vi "Drive at Angle.vi"(4 "end power":dbl, 6 "Begin power":dbl, 8 "error in (no error)":errorcluster, 9 "Angle":dbl, 10 "Distance":dbl, 11 "RobotDriveDevRef":T1={"DevStatus"={"status"=FALSE, "code"=0, "source"=""}, "Motors[]"=[], "Square Inputs"=FALSE, "Max Output"=1.0}) -> (0 "error out":errorcluster, 1 "power out":dbl, 3 "refnum":T1={"DevStatus"={"status"=FALSE, "code"=0, "source"=""}, "Motors[]"=[], "Square Inputs"=FALSE, "Max Output"=1.0})   [LabVIEW 2019]
uses:
  <vilib>/Rock Robotics/WPI/RobotDrive/WPI_RobotDriveArcadeDrive_Standard(NoSaturation).vi
  Infinite Recharge current/Robot Global Data.vi
  <vilib>/Rock Robotics/WPI/ThirdParty/Phoenix-LabVIEW/Motor Controller/Get/CTRE_Phoenix_MotorController_GetSelectedSensorData.vi
  <vilib>/Rock Robotics/SystemInterfaces/DIO/FPGA_DIOPWMChannel.ctl
  <vilib>/Rock Robotics/WPI/PWM/WPI_PWMDeadband.ctl
  <vilib>/Rock Robotics/WPI/MotorControl/WPI_MotorControlType.ctl
  <vilib>/Rock Robotics/SystemInterfaces/DIO/FPGA_DIOChannel.ctl
  <vilib>/Rock Robotics/WPI/MotorControl/WPI_MotorControlDeviceRef.ctl
  <vilib>/Rock Robotics/WPI/RobotDrive/WPI_RobotDriveDevRef.ctl
panel:
  out "error":dbl
  out "x/y":dbl
  out "Distance Left 2":dbl format="%#_13g"
  out "rampdown":dbl format="%#_13g"
  out "Maximup":dbl format="%#_13g"
  out "rampup":dbl format="%#_13g"
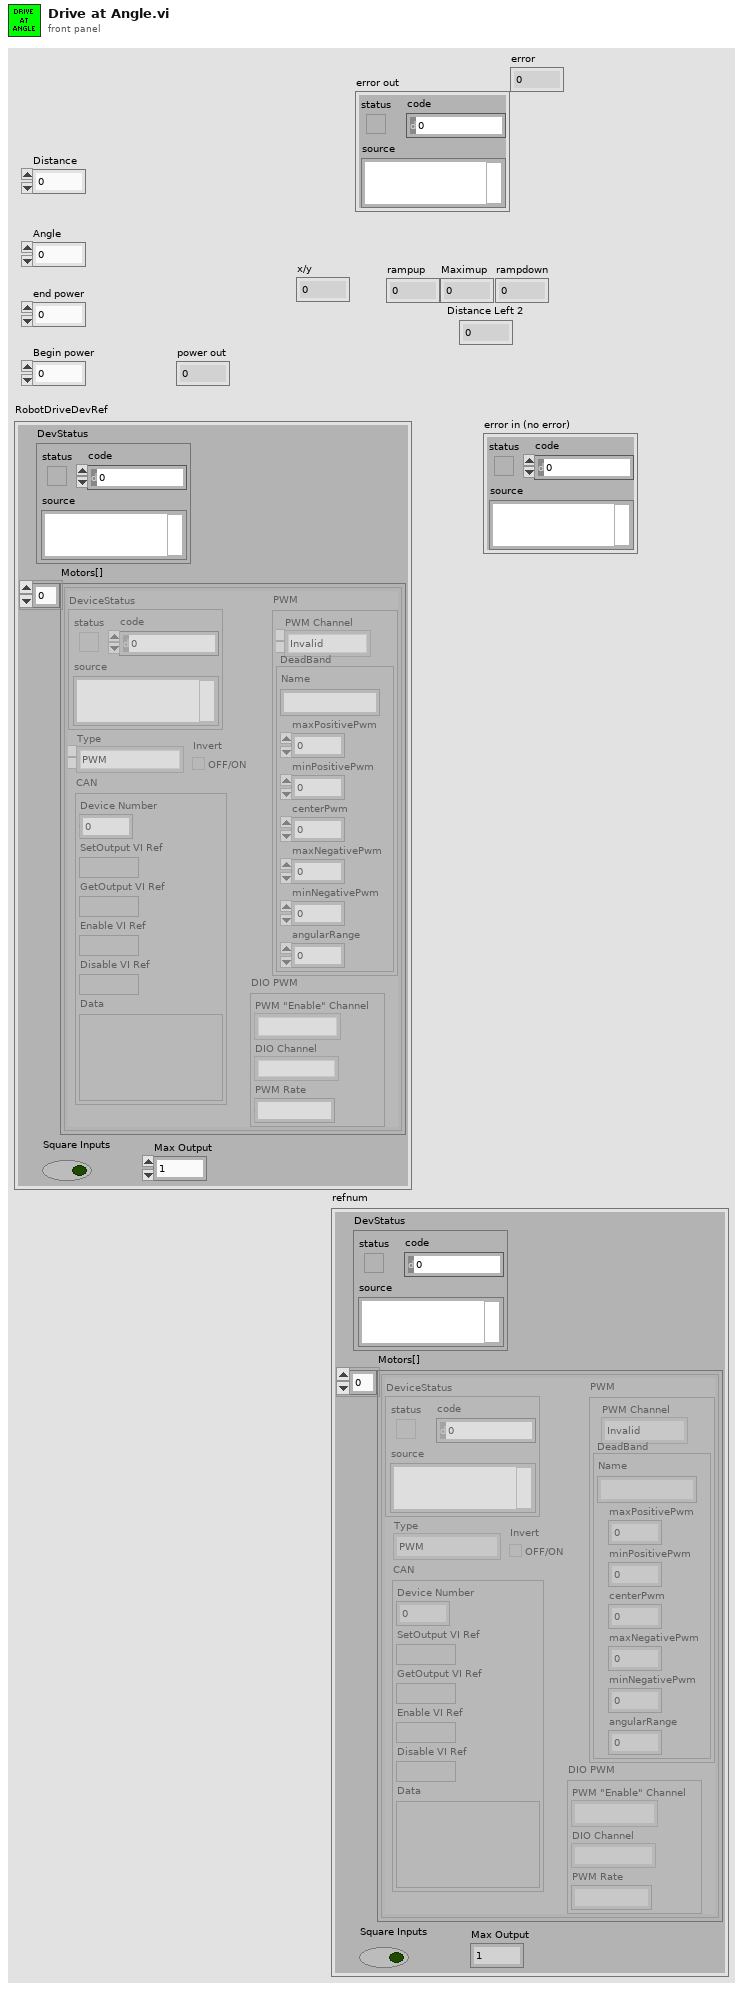
[diagram p1: front panel]
types:
  T1 = typedef "WPI_RobotDriveDevRef.ctl" = cluster{"DevStatus":errorcluster, "Motors[]":T2[], "Square Inputs":bool, "Max Output":dbl}
  T2 = typedef "WPI_MotorControlDeviceRef.ctl" = cluster{"DeviceStatus":errorcluster, "Type":T3, "PWM":cluster{"PWM Channel":T4, "DeadBand":T5}, "CAN":cluster{"Device Number":u8, "SetOutput VI Ref":variant, "GetOutput VI Ref":variant, "Enable VI Ref":variant, "Disable VI Ref":variant, "Data":variant}, "Invert":bool, "DIO PWM":cluster{"PWM \"Enable\" Channel":T4, "DIOChannel":T6, "PWM Rate":dbl}}
  T3 = typedef "WPI_MotorControlType.ctl" = enum16{"PWM", "CAN", "DIO PWM"}
  T4 = typedef "FPGA_DIOPWMChannel.ctl" = enum8{"PWM 0", "PWM 1", "PWM 2", "PWM 3", "PWM 4", "PWM 5", "PWM 6", "PWM 7", "PWM 8", "PWM 9", "PWM MXP 0", "PWM MXP 1", "PWM MXP 2", "PWM MXP 3", "PWM MXP 4", "PWM MXP 5", "PWM MXP 6", "PWM MXP 7", "PWM MXP 8", "PWM MXP 9", "Invalid"}
  T5 = typedef "WPI_PWMDeadband.ctl" = cluster{"Name":string, "maxPositivePwm":i32, "minPositivePwm":i32, "centerPwm":i32, "maxNegativePwm":i32, "minNegativePwm":i32, "angularRange":u16}
  T6 = typedef "FPGA_DIOChannel.ctl" = enum8{"DIO 0", "DIO 1", "DIO 2", "DIO 3", "DIO 4", "DIO 5", "DIO 6", "DIO 7", "DIO 8", "DIO 9", "DIO MXP 0", "DIO MXP 1", "DIO MXP 2", "DIO MXP 3", "DIO MXP 4", "DIO MXP 5", "DIO MXP 6", "DIO MXP 7", "DIO MXP 8", "DIO MXP 9", "DIO MXP 10", "DIO MXP 11", "DIO MXP 12", "DIO MXP 13", "DIO MXP 14", "DIO MXP 15", "SPI Port CS1", "SPI Port CS2", "SPI Port CS3", "SPI Port MISO", "SPI Port MOSI", "Invalid"}
  T7 = cluster{"Yaw":dbl, "Roll":dbl, "Pitch":dbl, "Heading":dbl, "Fused Heading":dbl}
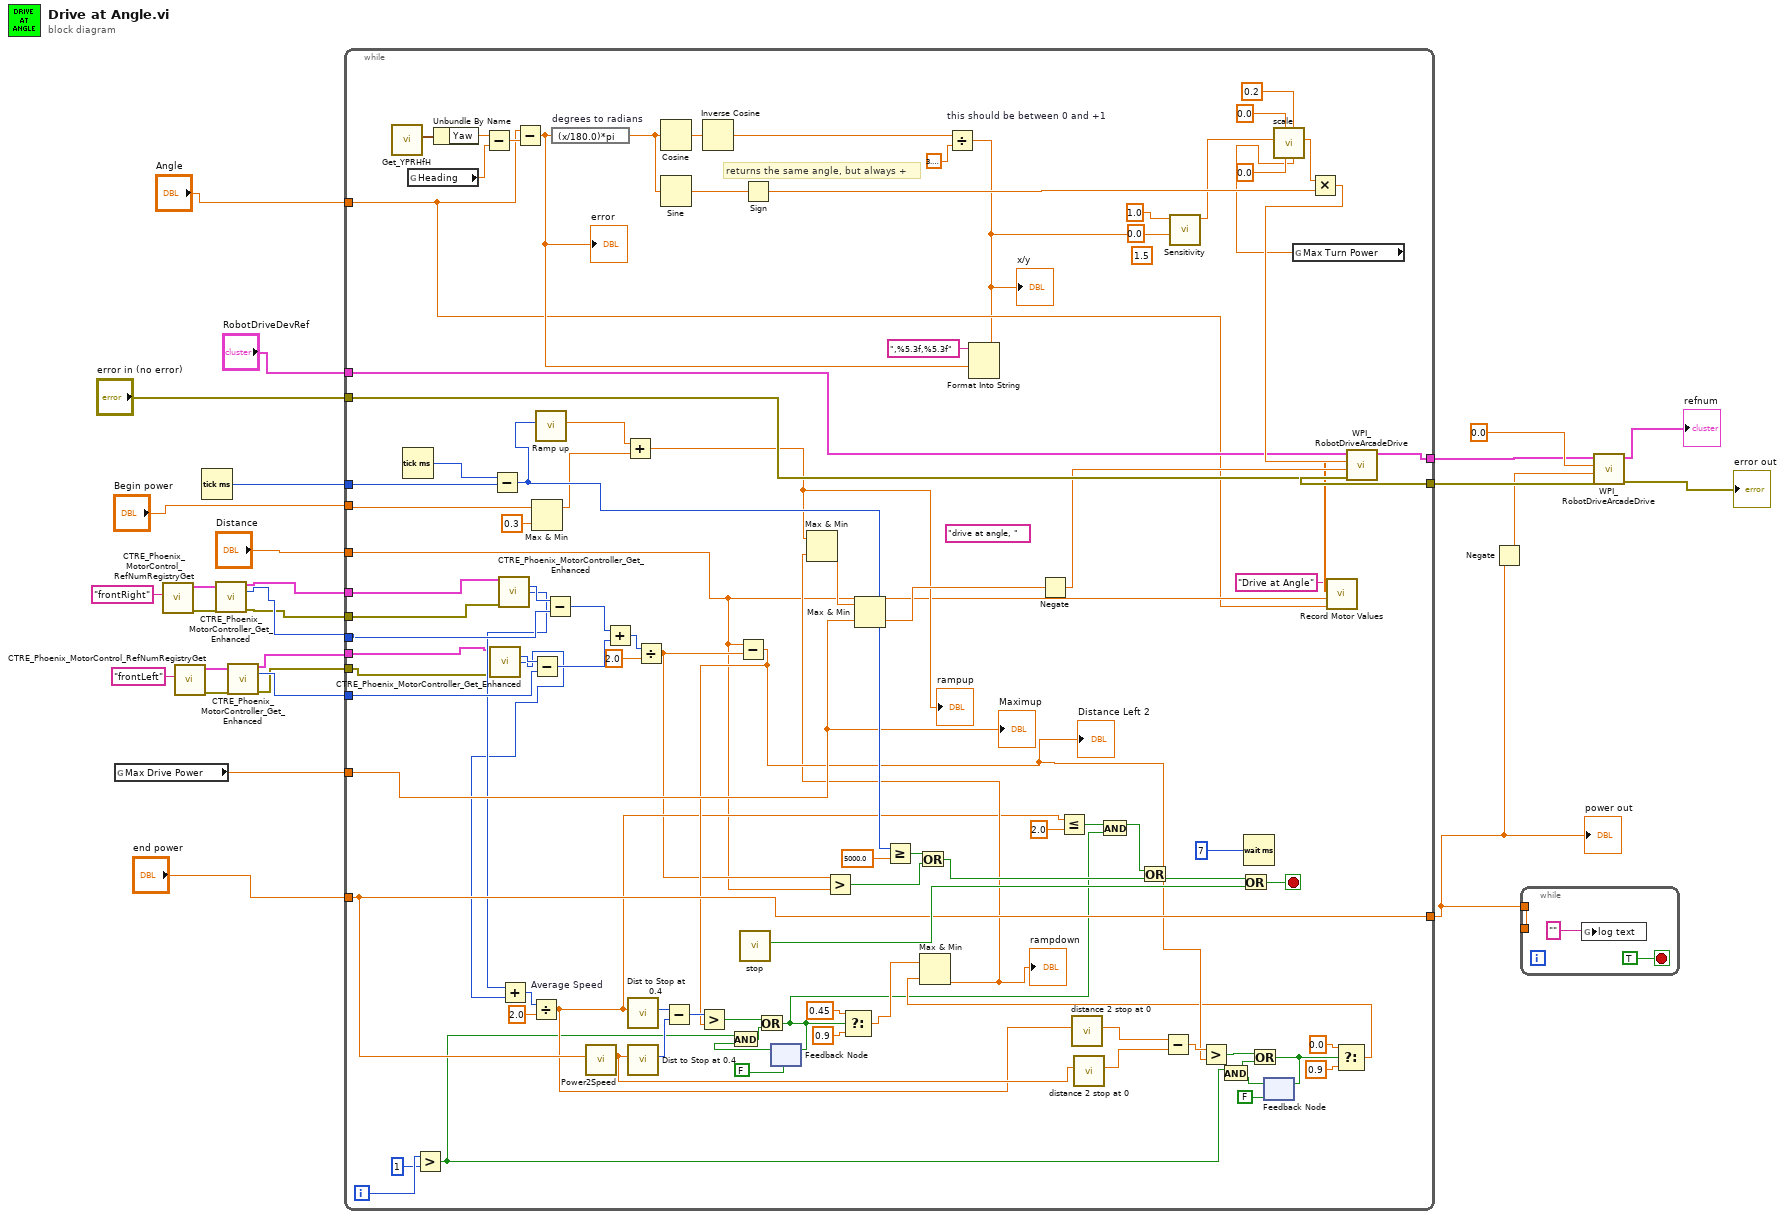
[diagram p0: block diagram]
diagram:
  n1 = global read "Robot Global Data.vi" "Max Drive Power"() -> (w15:dbl)
  n2 = call <vilib>:"CTRE_Phoenix_MotorControl_RefNumRegistryGet.vi"("refnum name"="frontRight") -> ("error out"=w7:errorcluster, "PhoenixMotorControlDevRef"=w8:T2)  [unwired: 9 in]
  n3 = call <vilib>:"CTRE_Phoenix_MotorControl_RefNumRegistryGet.vi"("refnum name"="frontLeft") -> ("error out"=w11:errorcluster, "PhoenixMotorControlDevRef"=w12:T2)  [unwired: 9 in]
  n4 = Tick Count (ms)() -> (millisecond timer value=w24:u32)
  n5 = call-poly <vilib>:"CTRE_Phoenix_MotorController_Get_Enhanced.vi"("PhoenixMotorControlDevRef"=w8, "error in"=w7) -> ("PhoenixMotorControlDevRef"=w4:T2, "Position (Raw Sensor Units)"=w5:i32, "error out"=w3:errorcluster)  [unwired: 10 in, 1 out]
  n6 = call-poly <vilib>:"CTRE_Phoenix_MotorController_Get_Enhanced.vi"("PhoenixMotorControlDevRef"=w12, "error in"=w11) -> ("PhoenixMotorControlDevRef"=w2:T2, "Position (Raw Sensor Units)"=w10:i32, "error out"=w1:errorcluster)  [unwired: 10 in, 1 out]
  n7 = while {
    tunnel: "Distance" -> [w44]
    tunnel: w5 -> [w125]
    tunnel: w10 -> [w126]
    tunnel: [w124] -> w26
    tunnel: [w123] -> w25
    tunnel: w4 -> [w35]
    tunnel: w3 -> [w32]
    tunnel: w2 -> [w31]
    tunnel: w24 -> [w117]
    tunnel: [w84] -> w13
    tunnel: "Angle" -> [w43]
    tunnel: "end power" -> [w84]
    tunnel: "RobotDriveDevRef" -> [w93]
    tunnel: "error in (no error)" -> [w92]
    tunnel: "Begin power" -> [w41]
    tunnel: w15 -> [w87]
    tunnel: w1 -> [w28]
    i -> [w54]
    stop <- w95 stop-if-true
    (unwired) 0.0 ("Low")
    (unwired) 1.5 ("Sensitivity")
    (unwired) "drive at angle, " ("string")
    # "returns the same angle, but always +"
    n8 = call <vilib>:"Get_YPRHfH.vi"() -> ("YRPHfH"=w115:T7)  [unwired: 11 in]
    n9 = Tick Count (ms)() -> (millisecond timer value=w116:u32)
    n10 = global read "Robot Global Data.vi" "Heading"() -> (w110:dbl)
    n11 = Greater?(x=w54, y=1) -> (0:w50:bool)
    n12 = Unbundle By Name(w115) -> ("Yaw"=w111:dbl)
    n13 = Subtract(x=w111, y=w110) -> (x-y=w109:dbl)
    n14 = call-poly <vilib>:"CTRE_Phoenix_MotorController_Get_Enhanced.vi"("PhoenixMotorControlDevRef"=w31, "error in"=w28) -> ("Position (Raw Sensor Units)"=w30:i32, "Velocity (Raw Sensor Units per 100 ms)"=w29:i32)  [unwired: 10 in, 2 out]
    n15 = Subtract(x=w116, y=w117) -> (x-y=w94:u32)
    n16 = call-poly <vilib>:"CTRE_Phoenix_MotorController_Get_Enhanced.vi"("PhoenixMotorControlDevRef"=w35, "error in"=w32) -> ("Position (Raw Sensor Units)"=w34:i32, "Velocity (Raw Sensor Units per 100 ms)"=w33:i32)  [unwired: 10 in, 2 out]
    n17 = Add(x=w33, y=w29) -> (x+y=w85:i32)
    n18 = Subtract(x=w43, y=w109) -> (x-y=w49:dbl)
    "error" <- w49
    n19 = Divide "Average Speed"(x=w85, y=2.0) -> (x/y=w58:dbl)
    n20 = Max & Min(x=w41, y=0.3) -> (max(x,y)=w42:dbl)  [unwired: 1 out]
    n21 = Subtract(x=w30, y=w126) -> (x-y=w119:i32)
    n22 = call "Ramp up.vi"("time"=w94) -> ("Power Out"=w91:dbl)  [unwired: 10 in]
    n23 = Subtract(x=w34, y=w125) -> (x-y=w120:i32)
    n24 = expression code="(x/180.0)*pi" "degrees to radians"(w49) -> (w112:dbl)
    n25 = call "Power2Speed.vi"("Power"=w84) -> ("Speed"=w73:dbl)  [unwired: 10 in]
    n26 = Add(x=w120, y=w119) -> (x+y=w122:i32)
    n27 = Add(x=w91, y=w42) -> (x+y=w88:dbl)
    "rampup" <- w88
    n28 = call "Dist to Stop at 0.4.vi"("Speed"=w58) -> ("Distance"=w83:i32)  [unwired: 10 in]
    n29 = call "Dist to Stop at 0.4.vi"("Speed"=w73) -> ("Distance"=w82:i32)  [unwired: 10 in]
    n30 = Divide(x=w122, y=2.0) -> (x/y=w55:dbl)
    n31 = Cosine(x=w112) -> (cos(x)=w114:dbl)
    n32 = Sine(x=w112) -> (sin(x)=w113:dbl)
    n33 = Subtract(x=w83, y=w82) -> (x-y=w81:i32)
    n34 = Inverse Cosine(1:w114) -> (0:w107:dbl)
    n35 = Subtract(x=w44, y=w55) -> (x-y=w71:dbl)
    "Distance Left 2" <- w71
    n36 = Greater?(x=w81, y=w71) -> (0:w80:bool)
    n37 = call "stop.vi"() -> ("Boolean"=w97:bool)  [unwired: 11 in]
    n38 = Sign(1:w113) -> (0:w102:dbl)
    n39 = feedback #1(FALSE) -> (w79:bool)
    n40 = And(x=w50, y=w79) -> (x .and. y?=w52:bool)
    n41 = Or(x=w80, y=w52) -> (x .or. y?=w56:bool)
    n42 = feedback-in #1(w56) -> ()
    n43 = Greater?(x=w55, y=w44) -> (0:w98:bool)
    n44 = Select(t=0.45, s=w56, f=0.9) -> (s? t:f=w63:dbl)
    n45 = Greater Or Equal?(x=w94, y=5000.0) -> (x >= y?=w99:bool)
    n46 = Or(x=w99, y=w98) -> (x .or. y?=w96:bool)
    n47 = Divide "this should be between 0 and +1"(x=w107, y=3.141592653589793) -> (x/y=w37:dbl)
    "x/y" <- w37
    n48 = Format Into String(initial string=",%5.3f,%5.3f", w49, w37) -> ()  [unwired: 2 in, 2 out]
    n49 = Less Or Equal?(x=w58, y=2.0) -> (x <= y?=w60:bool)
    n50 = call "distance 2 stop at 0.vi"("speed"=w58) -> ("Distance"=w75:dbl)  [unwired: 10 in]
    n51 = call "distance 2 stop at 0.vi"("speed"=w73) -> ("Distance"=w74:dbl)  [unwired: 10 in]
    n52 = And(x=w60, y=w56) -> (x .and. y?=w57:bool)
    n53 = Or(x=w57, y=w96) -> (x .or. y?=w61:bool)
    n54 = Subtract(x=w75, y=w74) -> (x-y=w72:dbl)
    n55 = call "Sensitivity.vi"("x"=w37, "sensitivity"=1.0 ("High")) -> ("scaled value"=w36:dbl)  [unwired: 9 in]
    n56 = Greater?(x=w72, y=w71) -> (0:w65:bool)
    n57 = Or(x=w61, y=w97) -> (x .or. y?=w95:bool)
    n58 = Wait (ms)(milliseconds to wait=u32 7) -> ()  [unwired: 1 out]
    n59 = feedback #2(FALSE) -> (w69:bool)
    n60 = And(x=w50, y=w69) -> (x .and. y?=w51:bool)
    n61 = Or(x=w65, y=w51) -> (x .or. y?=w70:bool)
    n62 = feedback-in #2(w70) -> ()
    n63 = global read "Robot Global Data.vi" "Max Turn Power"() -> (w39:dbl)
    n64 = call "scale.vi"("Max"=w39, "High"=0.2, "Min"=0.0, "Low"=0.0, "In Signal"=w36) -> ("Output signal"=w103:dbl)  [unwired: 6 in]
    n65 = Multiply(x=w103, y=w102) -> (x*y=w101:dbl)
    n66 = Select(t=0.0, s=w70, f=0.9) -> (s? t:f=w64:dbl)
    n67 = Max & Min(x=w63, y=w64) -> (min(x,y)=w62:dbl)  [unwired: 1 out]
    "rampdown" <- w62
    n68 = Max & Min(x=w88, y=w62) -> (min(x,y)=w90:dbl)  [unwired: 1 out]
    n69 = Max & Min(x=w90, y=w87) -> (min(x,y)=w89:dbl)  [unwired: 1 out]
    n70 = Negate(x=w89) -> (-x=w47:dbl)
    n71 = call-poly <vilib>:"WPI_RobotDriveArcadeDrive.vi"("error in (no error)"=w92, "Y axis value"=w47, "X axis value"=w101, "RobotDriveDevRef"=w93) -> ("error out"=w124:errorcluster, "Motor Values"=w46:dbl[], "RobotDriveDevRef"=w123:T1)  [unwired: 5 out]
    n72 = call "Record Motor Values.vi"("Target1 2"=w43, "Target1"=w44, "Motor Values"=w46, "VI Block Name"="Drive at Angle") -> ()  [unwired: 8 in]
    "Maximup" <- w87
  }
  "power out" <- w13
  n73 = Negate(x=w13) -> (-x=w14:dbl)
  n74 = while {
    tunnel: [w129] -> _
    tunnel: w13 -> [w129]
    stop <- TRUE stop-if-true
    n75 = global write "Robot Global Data.vi" "log text"("") -> ()
  }
  n76 = call-poly <vilib>:"WPI_RobotDriveArcadeDrive.vi"("error in (no error)"=w26, "Y axis value"=w14, "X axis value"=0.0, "RobotDriveDevRef"=w25) -> ("error out"=→"error out":errorcluster, "RobotDriveDevRef"=→"refnum":T1)  [unwired: 6 out]
